vi "MeasureJoule.vi"(5 "Junction Name":string, 6 "UiDefinition":T1, 7 ".NET Refnum":refnum<k24>, 8 "new file path (Not A Path if cancelled)":path, 10 "appended path":path, 11 ".NET Refnum in":refnum<k24>) -> (0 "error out":errorcluster, 3 "Cluster":cluster{dbl[], dbl[]})   [LabVIEW 2020]
uses:
  UIReferences.ctl
  C:/Users/User/Desktop/Automation/CurrentVersion/LabviewDXFViewer/bin/Release/LabviewDXFViewer.exe
  LabviewDXFViewer/bin/Release/LabviewDXFViewer.exe
  <vilib>/Utility/file.llb/Write Delimited Spreadsheet (DBL).vi
  <vilib>/Utility/file.llb/Write Delimited Spreadsheet (string).vi
panel:
  in  "CurrentPositionIndex":i32
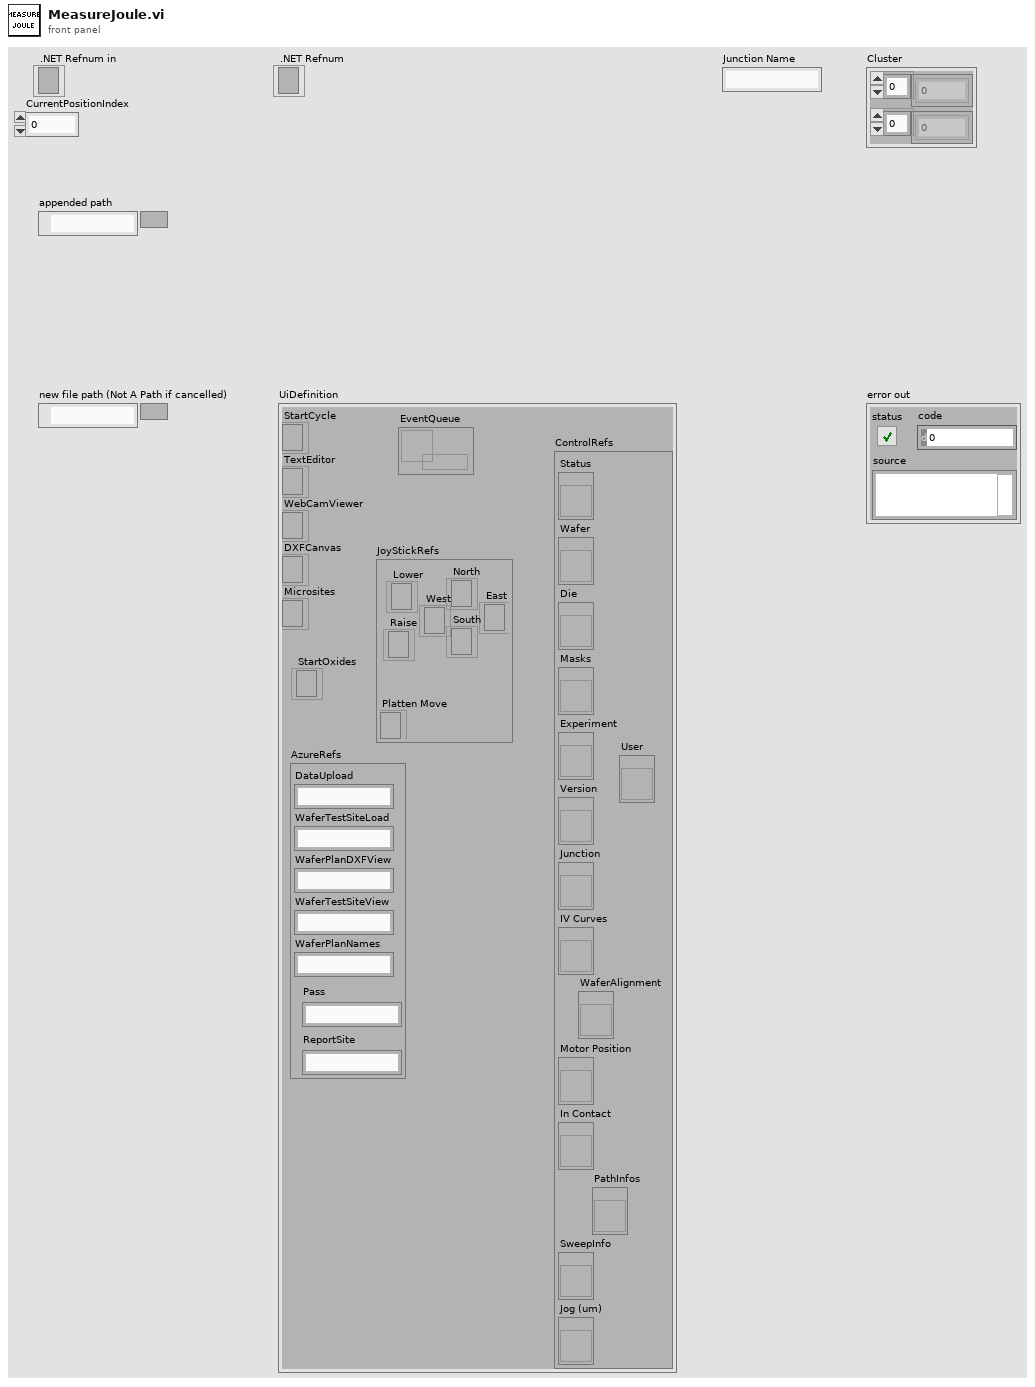
[diagram p1: front panel]
types:
  T1 = typedef "UIReferences.ctl" = cluster{"StartCycle":refnum<k24>, "TextEditor":refnum<k24>, "WebCamViewer":refnum<k24>, "DXFCanvas":refnum<k24>, "Microsites":refnum<k24>, "JoyStickRefs":cluster{"North":refnum<k24>, "Lower":refnum<k24>, "Raise":refnum<k24>, "Platten Move":refnum<k24>, "West":refnum<k24>, "East":refnum<k24>, "South":refnum<k24>}, "AzureRefs":cluster{"DataUpload":string, "WaferTestSiteLoad":string, "WaferPlanDXFView":string, "WaferTestSiteView":string, "WaferPlanNames":string, "Pass":string, "ReportSite":string}, "ControlRefs":cluster{"Status":refnum<vi>, "Wafer":refnum<vi>, "Die":refnum<vi>, "Masks":refnum<vi>, "Experiment":refnum<vi>, "Version":refnum<vi>, "Junction":refnum<vi>, "IV Curves":refnum<vi>, "Motor Position":refnum<vi>, "In Contact":refnum<vi>, "SweepInfo":refnum<vi>, "Jog (um)":refnum<vi>, "PathInfos":refnum<vi>, "User":refnum<vi>, "WaferAlignment":refnum<vi>}, "EventQueue":refnum<queue>, "StartOxides":refnum<k24>}
  T2 = typedef "CapacitanceInfos.ctl" = cluster{"Conductance":dbl, "CapacitanceIV":dbl, "Intercept":dbl, "CapacitanceSW":dbl, "Sum":dbl, "CapacitanceInfos":T3[], "CapacitancePhase":dbl, "dC/dV":dbl, "Function":string, "OtherInfo":dbl[][]}
  T3 = typedef "CapacitanceRecord.ctl" = cluster{"Freq":dbl, "Vpp":dbl, "PhaseS":dbl, "Irms":dbl, "PhaseC":dbl, "Theta":dbl, "VDrive":dbl, "Capacitance":dbl, "Other":dbl}
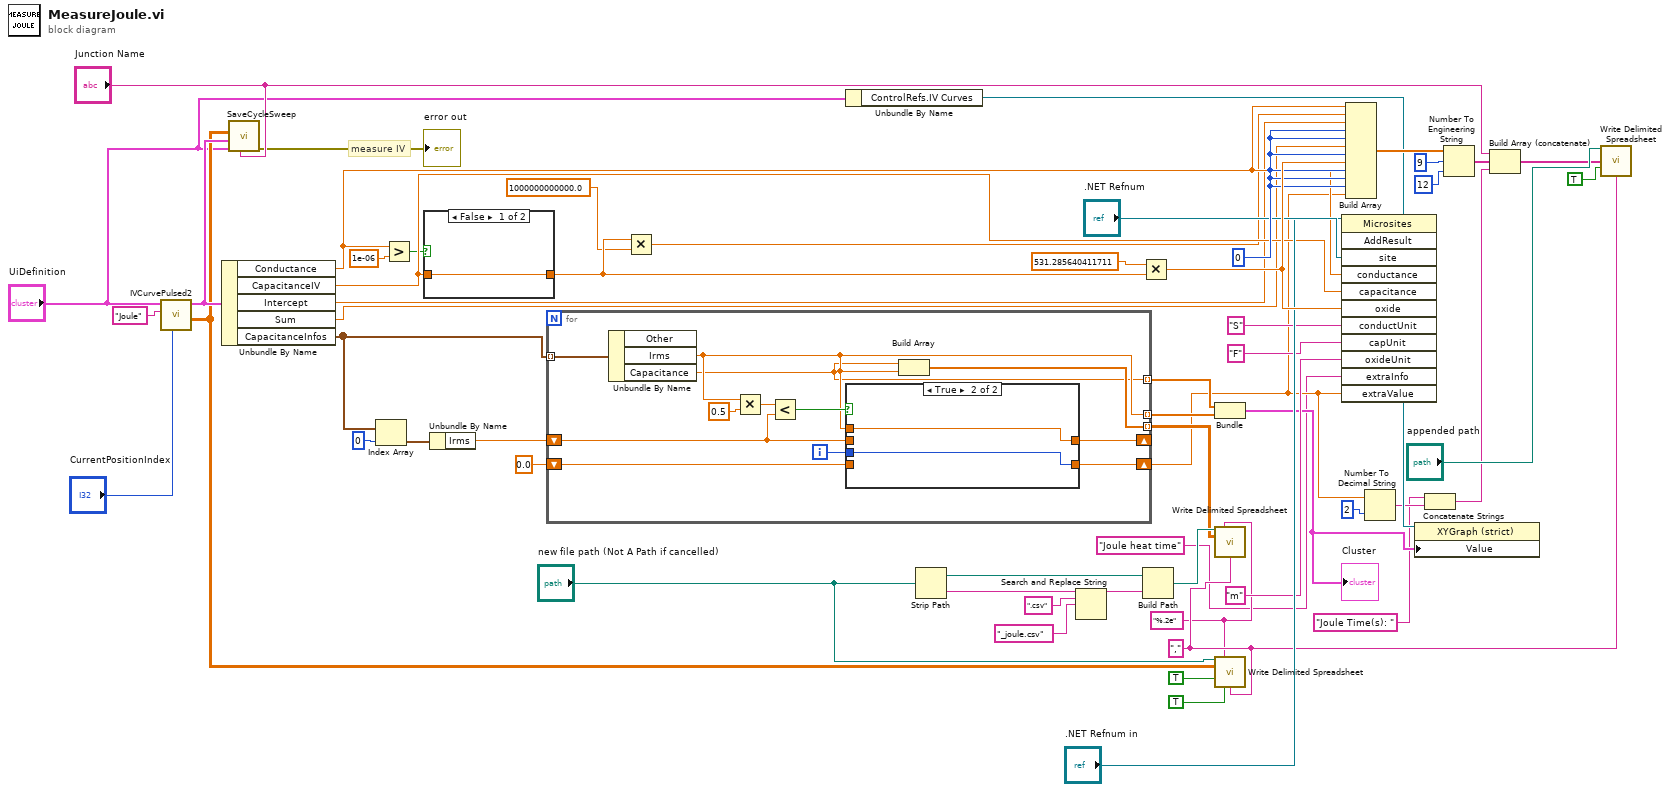
[diagram p0: block diagram]
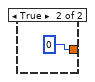
[diagram p3: hidden frame]
diagram:
  w12 = "," ("delimiter (\\t)")
  w55 = 0
  w11 = "%.2e" ("format (%.3f)")
  # "measure IV"
  n1 = call "IVCurvePulsed2.vi"("CurrentPositionIndex"="CurrentPositionIndex", "Program"="Joule", "UiDefinition"="UiDefinition") -> ("appended array"=w28:dbl[][], "InfoCluster"=w41:T2)  [unwired: 7 in]
  n2 = Unbundle By Name(w41) -> ("Conductance"=w43:dbl, "CapacitanceIV"=w42:dbl, "Intercept"=w31:dbl, "Sum"=w32:dbl, "CapacitanceInfos"=w46:T3[])
  n3 = call "SaveCycleSweep.vi"("JunctionName"="Junction Name", "UiDefinition 2"="UiDefinition", "InfoCluster"=w41, "appended array"=w28) -> ("error out"=→"error out":errorcluster)  [unwired: 7 in]
  n4 = Index Array(array=w46, index=0) -> (element=w48:T3)
  n5 = Greater?(x=w43, y=1e-06) -> (0:w35:bool)
  n6 = case shown="False" w35 {
    tunnel: [w59 0] -> w57
    tunnel: w42 -> [w59 _]
    frame False {
    }
    frame True {
    }
  }
  n7 = Unbundle By Name(w48) -> ("Irms"=w49:dbl)
  n8 = for {
    tunnel: w46 -> [w72] mode=indexing
    tunnel: [w61] -> w44 mode=indexing
    tunnel: [w63] -> w45 mode=indexing
    shift-right: [w65] -> _
    shift-left: w49 -> [w66]
    shift-right: [w70] -> w3
    shift-left: 0.0 ("Vpp") -> [w69]
    tunnel: [w62] -> w13 mode=indexing
    i -> [w64]
    n9 = Unbundle By Name(w72) -> ("Irms"=w63:dbl, "Capacitance"=w61:dbl)  [unwired: 1 out]
    n10 = Multiply(x=w63, y=0.5) -> (x*y=w68:dbl)
    n11 = Less?(x=w68, y=w66) -> (x < y?=w71:bool)
    n12 = case shown="True" w71 {
      tunnel: w64 -> [_ w76]
      tunnel: [w74 w76] -> w70
      tunnel: w69 -> [w74 _]
      tunnel: [w73 w75] -> w65
      tunnel: w66 -> [w73 _]
      tunnel: w63 -> [_ w75]
      frame False {
      }
      frame True {
      }
    }
    n13 = Build Array(w61, w63) -> (w62:dbl[])
  }
  n14 = Multiply(x=w57, y=1000000000000.0) -> (x*y=w33:dbl)
  n15 = Unbundle By Name("UiDefinition") -> ("ControlRefs.IV Curves"=w9:refnum<vi>)
  n16 = Strip Path(path="new file path (Not A Path if cancelled)") -> (stripped path=w16:path, name=w20:string)
  n17 = Search and Replace String(input string=w20, search string=".csv", replace string="_joule.csv" ("replace string (\"\")")) -> (result string=w17:string)  [unwired: 5 in, 3 out]
  n18 = Multiply(x=531.285640411711, y=w57) -> (x*y=w58:dbl)
  n19 = Build Path(base path=w16, name or relative path=w17) -> (appended path=w14:path)
  n20 = Bundle(w44, w45) -> (w8:cluster{dbl[], dbl[]})  [unwired: 1 in]
  "Cluster" <- w8
  n21 = call-poly <vilib>:"Write Delimited Spreadsheet.vi"("file path (dialog if empty)"=w14, "format (%.3f)"=w11, "2D data"=w13, "delimiter (\\t)"=w12) -> ()  [unwired: 10 in, 2 out]
  n22 = call-poly <vilib>:"Write Delimited Spreadsheet.vi"("file path (dialog if empty)"="new file path (Not A Path if cancelled)", "format (%.3f)"=w11, "2D data"=w28, "append to file? (new file:F)"=TRUE, "transpose? (no:F)"=TRUE, "delimiter (\\t)"=w12) -> ()  [unwired: 8 in, 2 out]
  n23 = invoke class="Microsites" method="AddResult"(reference=".NET Refnum in", "site"=".NET Refnum", "conductance"=w43, "capacitance"=w42, "oxide"=w58, "conductUnit"="S", "capUnit"="F", "oxideUnit"="m" ("interceptUnit"), "extraInfo"="Joule heat time", "extraValue"=w3) -> ()  [unwired: 2 in, 12 out]
  n24 = Build Array(w43, w33, w31, w55, w55, w32, w55, w58, w55, w55, w55, w3) -> (w30:dbl[])
  n25 = Number To Decimal String(number=w3, width (-)=i16 2) -> (decimal integer string=w7:string)
  n26 = property class="XYGraph (strict)"(reference=w9, "Value"=w8) -> ()  [unwired: 1 in, 2 out]
  n27 = Concatenate Strings("Joule Time(s): ", w7) -> (w4:string)
  n28 = Number To Engineering String(2:i16 12 ("precision (6)"), 3:i16 9 ("width (-)"), 4:w30) -> (0:w23:string[])  [unwired: 1 in]
  n29 = Build Array (concatenate)("Junction Name", w23, w4) -> (w25:string[])
  n30 = call-poly <vilib>:"Write Delimited Spreadsheet.vi"("file path (dialog if empty)"="appended path", "1D data"=w25, "append to file? (new file:F)"=TRUE, "delimiter (\\t)"=w12) -> ()  [unwired: 10 in, 2 out]
